vi "VR-init.vi"(8 "error in (no error)":errorcluster, 11 "VR-VNA_root in":refnum<class "VR-VNA_root.lvclass">) -> (0 "error out":errorcluster, 3 "VR-VNA_root out":refnum<class "VR-VNA_root.lvclass">)   [LabVIEW 2020, in "VR-VNA_root.lvlib" / "VR-VNA_root.lvclass"]
uses:
  VR-VNA_root.lvclass
  VR-VNA_root.lvclass/VR-VNA_root.ctl
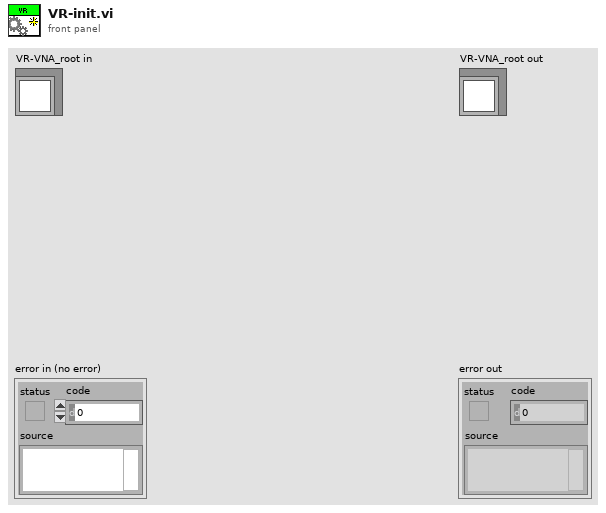
[diagram p1: front panel]
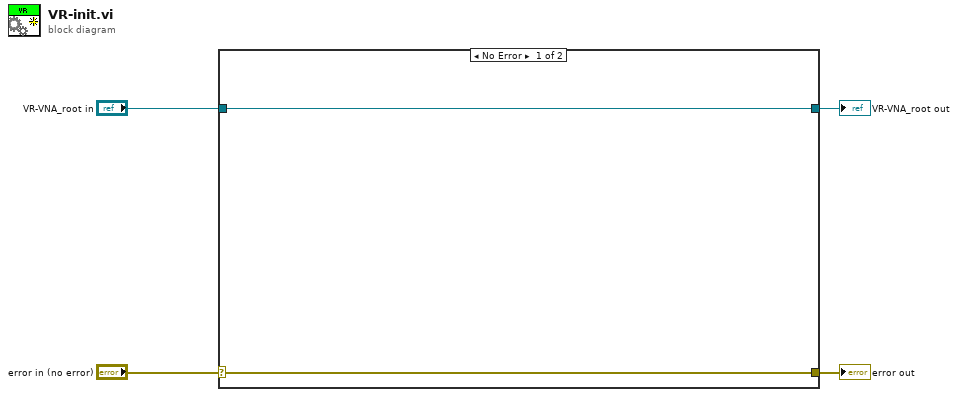
[diagram p0: block diagram]
diagram:
  n1 = case shown="No Error" "error in (no error)" {
    selector: "error in (no error)" -> [w5 w8]
    tunnel: [w5 w8] -> w3
    tunnel: [w6 w7] -> w1
    tunnel: "VR-VNA_root in" -> [w6 w7]
    frame No Error {
    }
    frame Error {
    }
  }
  "error out" <- w3
  "VR-VNA_root out" <- w1
